vi "Handle UNSUBSCRIBED.vi"(8 "error in (no error)":errorcluster, 9 "Message Loop data (in)":T1, 10 "WAMP Message":T16 {"Message Codes" items=["HELLO"=1, "WELCOME"=2, "ABORT"=3, "GOODBYE"=6, "ERROR"=8, "PUBLISH"=16, "PUBLISHED"=17, "SUBSCRIBE"=32, "SUBSCRIBED"=33, "UNSUBSCRIBE"=34, "UNSUBSCRIBED"=35, "EVENT"=36, "CALL"=48, "RESULT"=59, "REGISTER"=64, "REGISTERED"=65, "UNREGISTER"=66, "UNREGISTERED"=67, "INVOCATION"=68, "YIELD"=70]}, 11 "reference":refnum<class "WAMP Client.lvclass">) -> (0 "error out":errorcluster, 1 "Message Loop Data (Out)":T1, 3 "reference out":refnum<class "WAMP Client.lvclass">)   [LabVIEW 2020, in "wamplv.lvlib" / "WAMP Client.lvclass"]
uses:
  WAMP Client.lvclass
  TypeDef/WAMP Received Message.ctl
  TypeDef/WAMP Message Codes.ctl
  TypeDef/Message Loop Data.ctl
  TypeDef/REGISTER Request Data.ctl
  TypeDef/Success or error.ctl
  API/TypeDefs/Combined error.ctl
  API/TypeDefs/WAMP error.ctl
  TypeDef/Publish Requests Map.ctl
  TypeDef/PUBLISH Request Data.ctl
  TypeDef/PUBLISH result.ctl
  TypeDef/Endpoint Data.ctl
  TypeDef/CALL Request Map.ctl
  TypeDef/CALL Request Data.ctl
  API/TypeDefs/RESULT payload.ctl
  TypeDef/SUBSCRIBE Requests Map.ctl
  TypeDef/SUBSCRIBE Request Data.ctl
  TypeDef/Subscribe Result.ctl
  TypeDef/EVENT payload.ctl
  TypeDef/Subscriptions Map.ctl
  TypeDef/Subscription Details.ctl
  TypeDef/Unsubscribe Requests Map.ctl
  TypeDef/UNSUBSCRIBE Request Data.ctl
  TypeDef/UNSUBSCRIBE Result.ctl
  TypeDef/Unregister requests map.ctl
  TypeDef/Unregister request.ctl
  a6a1983e-7ce6-4ada-aacc-f5172fec86f2.vi
  a3bfe72d-438f-42b9-9e71-0b3ebc88a09d.vi
  73a204a7-fc9f-47f9-93b3-f48d89583bd3.vi
  <vilib>/Utility/error.llb/Error Cluster From Error Code.vi
  WAMP Client.lvclass/WAMP Client.ctl
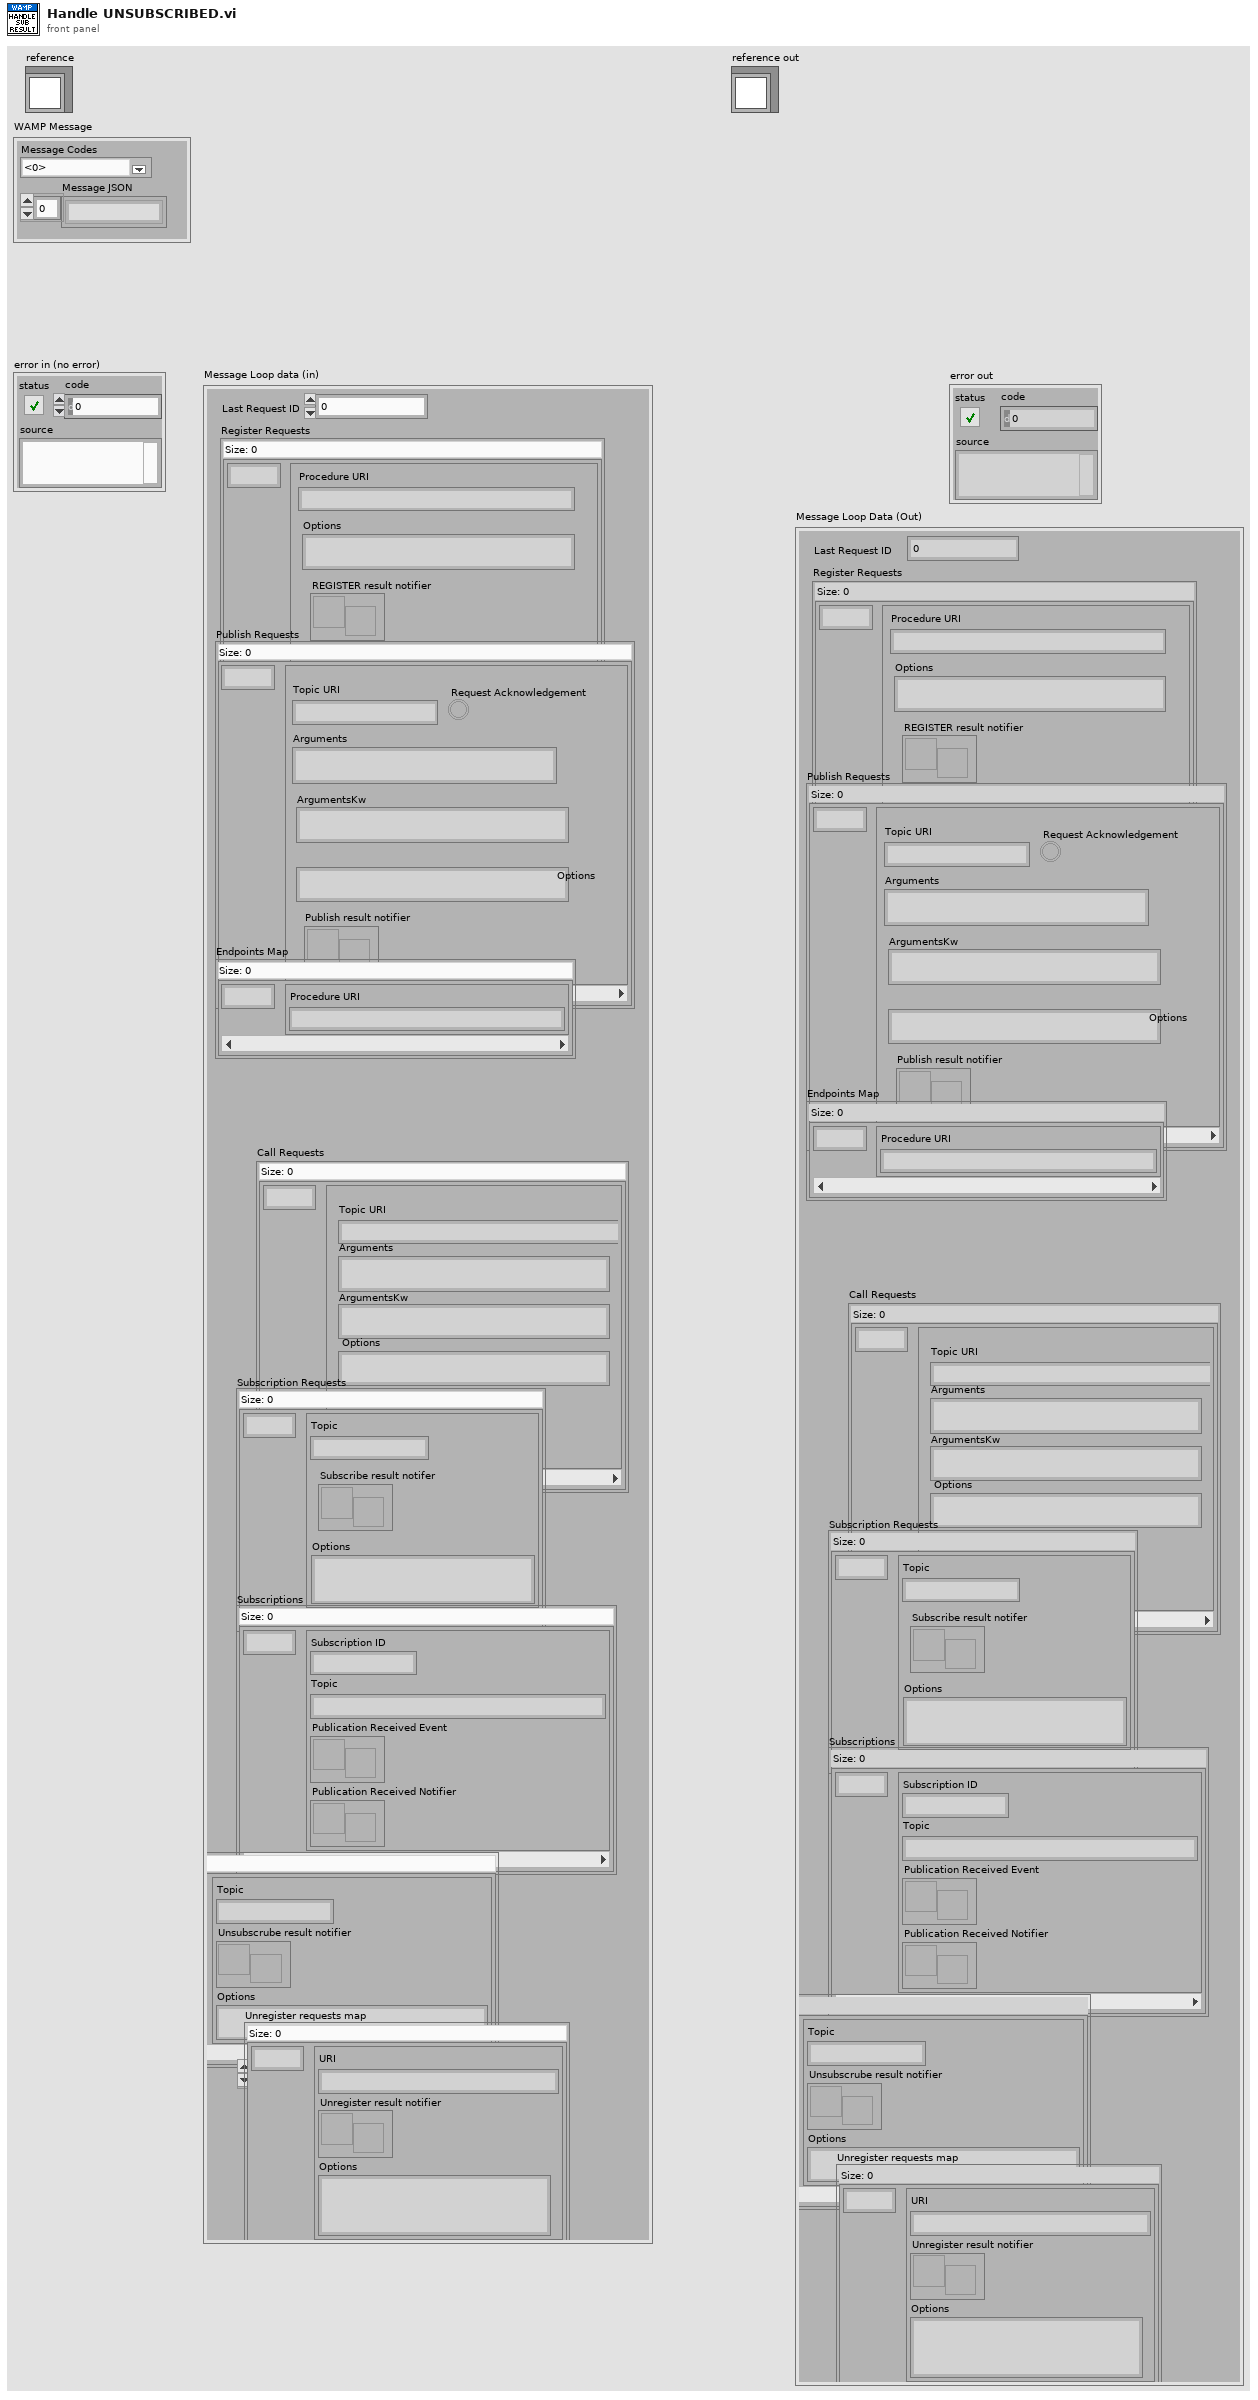
[diagram p1: front panel]
types:
  T1 = typedef "wamplv.lvlib/WAMP Client.lvclass/Message Loop Data.ctl" = cluster{"Last Request ID":u64, "Register Requests":map{u64, T2}, "Publish Requests":T3, "Endpoints Map":map{u64, T5}, "Call Requests":T6, "Subscription Requests":T8, "Subscriptions":T10, "Unsubscribe Requests":T12, "Random Request IDs":u64[], "Unregister requests map":T14}
  T2 = typedef "wamplv.lvlib/WAMP Client.lvclass/REGISTER Request Data.ctl" = cluster{"Procedure URI":string, "Options":string, "REGISTER result notifier":refnum<notifier>}
  T3 = typedef "wamplv.lvlib/WAMP Client.lvclass/Publish Requests Map.ctl" = map{u64, T4}
  T4 = typedef "wamplv.lvlib/WAMP Client.lvclass/PUBLISH Request Data.ctl" = cluster{"Topic URI":string, "Arguments":string, "ArgumentsKw":string, "Request Acknowledgement":bool, "Options":string, "Publish result notifier":refnum<notifier>}
  T5 = typedef "wamplv.lvlib/WAMP Client.lvclass/Endpoint Data.ctl" = cluster{"Procedure URI":string}
  T6 = typedef "wamplv.lvlib/WAMP Client.lvclass/CALL Request Map.ctl" = map{u64, T7}
  T7 = typedef "wamplv.lvlib/WAMP Client.lvclass/CALL Request Data.ctl" = cluster{"Topic URI":string, "Arguments":string, "ArgumentsKw":string, "Options":string, "Call result":refnum<notifier>}
  T8 = typedef "wamplv.lvlib/WAMP Client.lvclass/SUBSCRIBE Requests Map.ctl" = map{u64, T9}
  T9 = typedef "wamplv.lvlib/WAMP Client.lvclass/SUBSCRIBE Request Data.ctl" = cluster{"Topic":string, "Subscribe result notifer":refnum<notifier>, "Options":string}
  T10 = typedef "wamplv.lvlib/WAMP Client.lvclass/Subscriptions Map.ctl" = map{u64, T11}
  T11 = typedef "wamplv.lvlib/WAMP Client.lvclass/Subscription Details.ctl" = cluster{"Subscription ID":u64, "Topic":string, "Publication Received Event":refnum<user-event>, "Publication Received Notifier":refnum<notifier>}
  T12 = typedef "wamplv.lvlib/WAMP Client.lvclass/Unsubscribe Requests Map.ctl" = map{u64, T13}
  T13 = typedef "wamplv.lvlib/WAMP Client.lvclass/UNSUBSCRIBE Request Data.ctl" = cluster{"Topic":string, "Unsubscrube result notifier":refnum<notifier>, "Options":string}
  T14 = typedef "wamplv.lvlib/WAMP Client.lvclass/Unregister requests map.ctl" = map{u64, T15}
  T15 = typedef "wamplv.lvlib/WAMP Client.lvclass/Unregister request.ctl" = cluster{"URI":string, "Unregister result notifier":refnum<notifier>, "Options":string}
  T16 = typedef "wamplv.lvlib/WAMP Client.lvclass/WAMP Received Message.ctl" = cluster{"Message JSON":string[], "Message Codes":T17}
  T17 = typedef "wamplv.lvlib/WAMP Client.lvclass/WAMP Message Codes.ctl" = u16
  T18 = typedef "wamplv.lvlib/WAMP Client.lvclass/UNSUBSCRIBE Result.ctl" = cluster{"Success?":bool, "Combined Error":T19}
  T19 = typedef "wamplv.lvlib/WAMP Client.lvclass/Combined error.ctl" = cluster{"Error?":bool, "WAMP Error":T20, "Error":errorcluster}
  T20 = typedef "wamplv.lvlib/WAMP Client.lvclass/WAMP error.ctl" = cluster{"Details":string, "ArgumentKw Payload":string, "Error?":bool, "Error URI":string, "Arguments Payload":string}
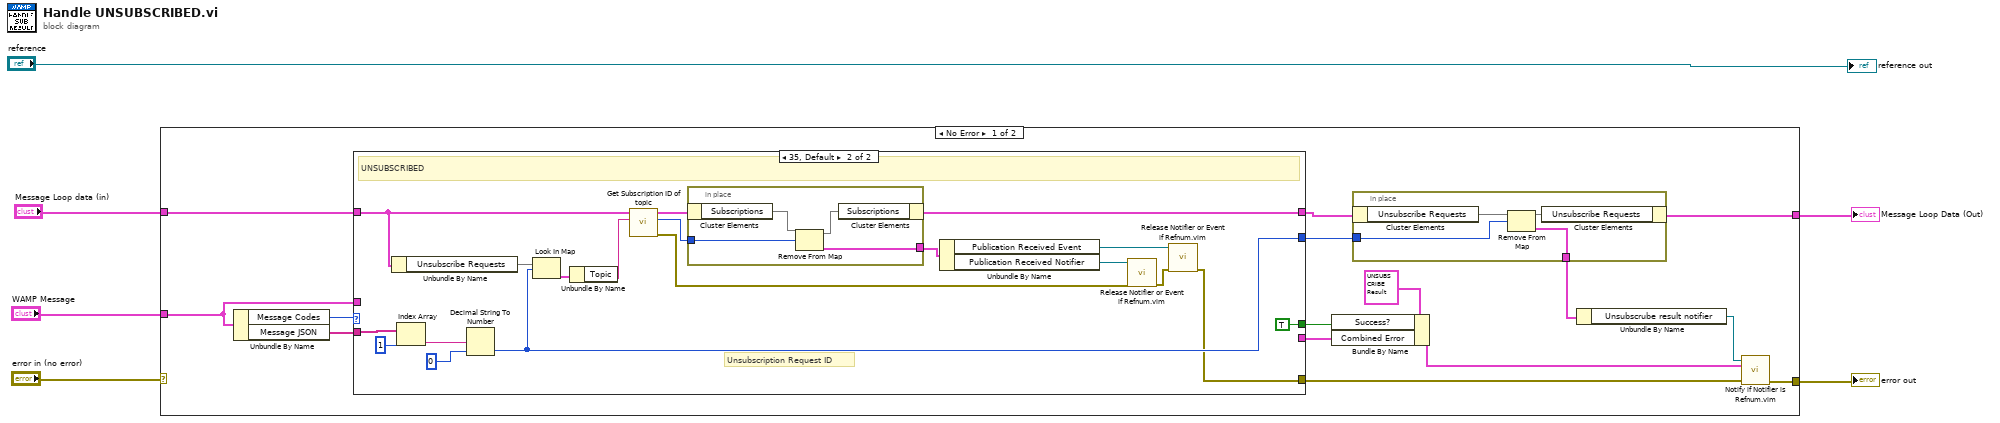
[diagram p0: block diagram]
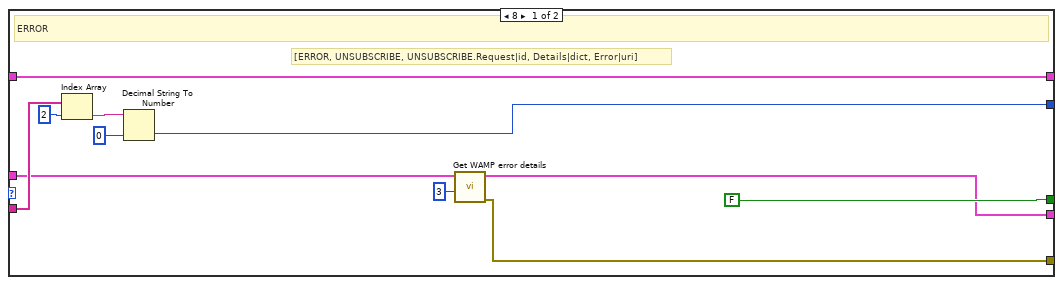
[diagram p2: hidden frame]
diagram:
  n1 = case shown="No Error" "error in (no error)" {
    selector: "error in (no error)" -> [_ w60]
    tunnel: "Message Loop data (in)" -> [w14 w61]
    tunnel: "WAMP Message" -> [w13 _]
    tunnel: [w9 w60] -> w2
    tunnel: [w7 w61] -> w1
    frame No Error {
      n2 = Unbundle By Name(w13) -> ("Message Codes"=w19:T17, "Message JSON"=w18:string[])
      n3 = case shown="35, Default" w19 {
        tunnel: w18 -> [w34 w51]
        tunnel: [w33 w49] -> w17
        tunnel: [w26 w37] -> w12
        tunnel: [w27 _] -> w21
        tunnel: [FALSE ("Success?") TRUE ("Success?")] -> w20
        tunnel: w14 -> [w32 w46]
        tunnel: [w32 w43] -> w8
        tunnel: w13 -> [w29 _]
        frame 8 {
          # "[ERROR, UNSUBSCRIBE, UNSUBSCRIBE.Request|id, Details|dict, Error|uri]"
          # "ERROR"
          n4 = Index Array(array=w34, index=2) -> (element=w35:string)
          n5 = Decimal String To Number(string=w35, default (0L)=u64 0 ("default (0 I32)")) -> (number=w33:u64)  [unwired: 1 in, 1 out]
          n6 = call "Get WAMP error details.vi"("Details Index"=u32 3, "WAMP Message"=w29) -> ("error out"=w26:errorcluster, "Combined Error"=w27:T19)  [unwired: 7 in, 1 out]
        }
        frame 35, Default {
          # "Unsubscription Request ID"
          # "UNSUBSCRIBED"
          n7 = Unbundle By Name(w46) -> ("Unsubscribe Requests"=w50:T12)
          n8 = Index Array(array=w51, index=1) -> (element=w53:string)
          n9 = Decimal String To Number(string=w53, default (0L)=u64 0) -> (number=w49:u64)  [unwired: 1 in, 1 out]
          n10 = Look In Map(map=w50, key=w49) -> (value=w48:T13)  [unwired: 1 in, 1 out]
          n11 = Unbundle By Name(w48) -> ("Topic"=w47:string)
          n12 = call "Get Subscription ID of topic.vi"("Topic"=w47, "Message loop data (in)"=w46) -> ("error out"=w38:errorcluster, "Subscription ID"=w45:u64, "Message loop data (out)"=w44:T1)  [unwired: 7 in]
          n13 = in-place {
            in-place-border: w45 -> [w59]
            in-place-border: [w56] -> w42
            n14 = in-place-cluster #1(w44) -> ("Subscriptions"=w58:T10)
            n15 = Remove From Map(10:w59, 11:w58) -> (1:w56:T11, 3:w57:T10)  [unwired: 1 out]
            n16 = in-place-cluster #1("Subscriptions"=w57) -> (w43:T1)
          }
          n17 = Unbundle By Name(w42) -> ("Publication Received Event"=w40:refnum<user-event>, "Publication Received Notifier"=w41:refnum<notifier>)
          n18 = call "Release Notifier or Event if Refnum.vim"("error in (no error)"=w38, "Notifier or Event in"=w41) -> ("error out"=w39:errorcluster)  [unwired: 9 in]
          n19 = call "Release Notifier or Event if Refnum.vim"("error in (no error)"=w39, "Notifier or Event in"=w40) -> ("error out"=w37:errorcluster)  [unwired: 9 in]
        }
      }
      n20 = Bundle By Name(cluster=T18 {"Success?"=FALSE, "Combined Error"={"Error?"=FALSE, "WAMP Error"={"Details"="", "ArgumentKw Payload"="{}", "Error?"=FALSE, "Error URI"="", "Arguments Payload"=""}, "Error"={"status"=FALSE, "code"=0, "source"=""}}} ("Unsubcsribe Result"), "Success?"=w20, "Combined Error"=w21) -> (w11:T18)
      n21 = in-place "In Place Element Structure" {
        in-place-border: w17 -> [w25]
        in-place-border: [w24] -> w16
        n22 = in-place-cluster #2(w8) -> ("Unsubscribe Requests"=w23:T12)
        n23 = Remove From Map(10:w25, 11:w23) -> (1:w24:T13, 3:w22:T12)  [unwired: 1 out]
        n24 = in-place-cluster #2("Unsubscribe Requests"=w22) -> (w7:T1)
      }
      n25 = Unbundle By Name(w16) -> ("Unsubscrube result notifier"=w10:refnum<notifier>)
      n26 = call "Notify if Notifier is Refnum.vim"("error in (no error)"=w12, "RESULT Payload"=w11, "Notifier in"=w10) -> ("error out"=w9:errorcluster)  [unwired: 8 in]
    }
    frame Error {
    }
  }
  "error out" <- w2
  "Message Loop Data (Out)" <- w1
  "reference out" <- "reference"
